vi "测试-循环输入给python程序.vi"() -> ()   [LabVIEW 2018]
panel:
  in  "关闭界面":bool
  out "图片/视频路径":string
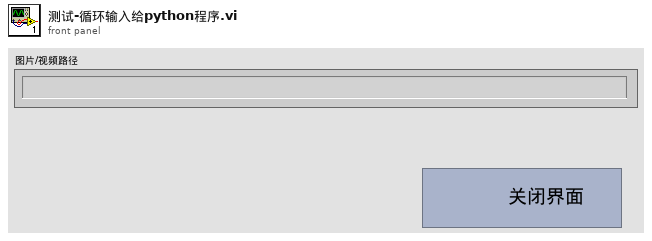
[diagram p1: front panel]
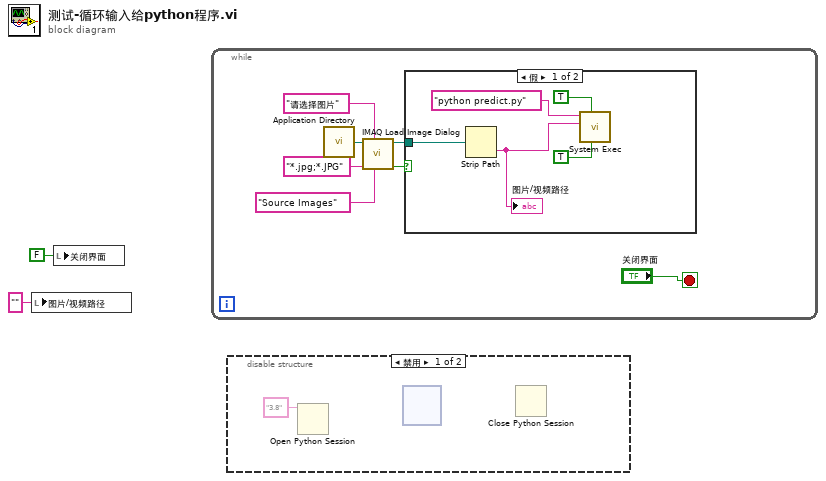
[diagram p0: block diagram]
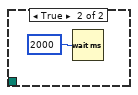
[diagram p3: hidden frame]
diagram:
  n1 = local write "图片/视频路径"("" ("图片/视频路径")) -> ()
  n2 = local write "关闭界面"(FALSE ("关闭界面")) -> ()
  n3 = while {
    stop <- "关闭界面" stop-if-true
    n4 = call <vilib>:"Application Directory.vi"() -> ("Application Directory"=w8:path)
    n5 = call "IMAQ Load Image Dialog"("Pattern Label"="Source Images", "Prompt"="请选择图片" ("prompt"), "Pattern"="*.jpg;*.JPG", "Start Path"=w8) -> ("Cancelled?"=w4:bool, "Path"=w3:path)  [unwired: 5 in, 1 out]
    n6 = case shown="假" w4 {
      tunnel: w3 -> [w10 _]
      frame False {
        n7 = Strip Path(path=w10) -> (name=w14:string)  [unwired: 1 out]
        "图片/视频路径" <- w14
        n8 = call <vilib>:"System Exec.vi"("run minimized? (F)"=TRUE, "wait until completion? (T)"=TRUE, "standard input"=w14, "command line"="python predict.py") -> ()  [unwired: 4 in, 4 out]
      }
      frame True {
        n9 = Wait (ms)(milliseconds to wait=u32 2000 ("等待时间（毫秒）")) -> ()  [unwired: 1 out]
      }
    }
  }
  n10 = disable-structure shown="禁用" {
    frame Disabled {
      n11 = Open Python Session(python version="3.8" ("Python版本")) -> ()  [unwired: 2 in, 2 out]
      n12 = node() -> ()  [unwired: 6 in, 4 out]
      n13 = Close Python Session() -> ()  [unwired: 2 in, 1 out]
    }
    frame Enabled {
    }
  }
